vi "Create.vi"(8 "error in (no error)":errorcluster, 10 "Append Index (-1)":i32=-1, 11 "File Type":T1) -> (0 "error out":errorcluster, 3 "Data out":refnum<class "Data.lvclass">)   [LabVIEW 2019, in "Data.lvclass"]
uses:
  Data.lvclass
  Data.DAT/Data.DAT.lvclass
  Data.ITX/Data.ITX.lvclass
  Data.TDMS/Data.TDMS.lvclass
  Typedefs/File Type--enum.ctl
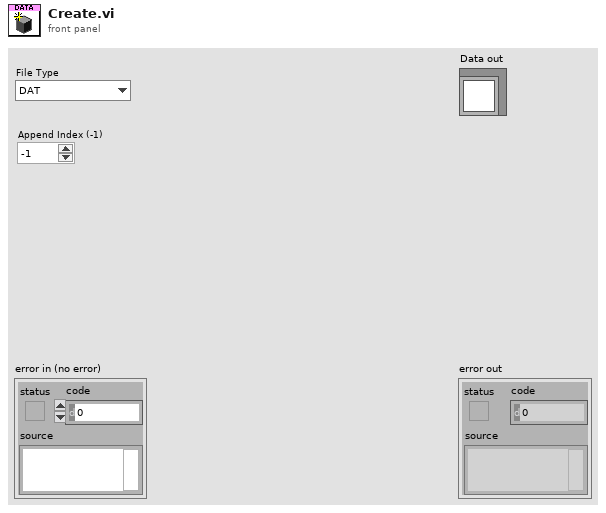
[diagram p1: front panel]
types:
  T1 = typedef "Data.lvclass/File Type--enum.ctl" = enum16{"DAT", "ITX", "TDMS", "VI"}
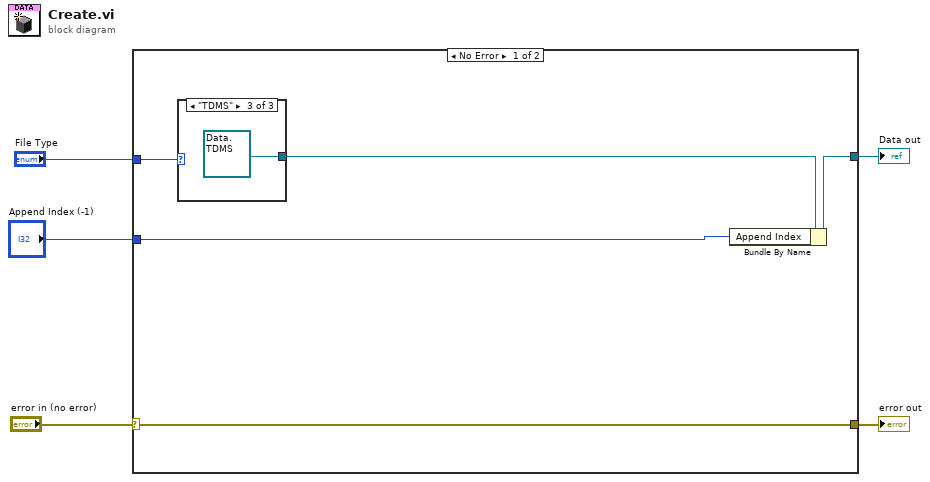
[diagram p0: block diagram]
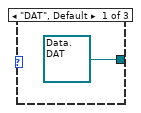
[diagram p2: hidden frame]
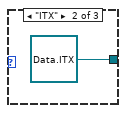
[diagram p3: hidden frame]
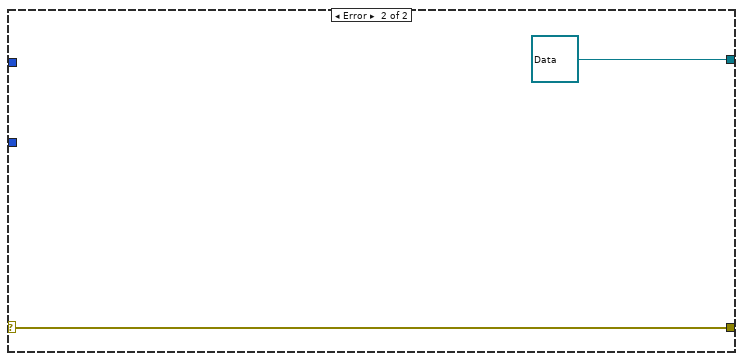
[diagram p4: hidden frame]
diagram:
  n1 = case shown="No Error" "error in (no error)" {
    selector: "error in (no error)" -> [w10 w15]
    tunnel: [w10 w15] -> w4
    tunnel: [w7 refnum<class "Data.lvclass"> refnum ("ITX")] -> w3
    tunnel: "File Type" -> [w9 _]
    tunnel: "Append Index (-1)" -> [w6 _]
    frame No Error {
      n2 = case shown="\"TDMS\"" w9 {
        tunnel: [refnum<class "Data.DAT.lvclass"> refnum ("DAT.lvclass") refnum<class "Data.ITX.lvclass"> refnum ("ITX") refnum<class "Data.TDMS.lvclass"> refnum ("Data.TDMS.lvclass")] -> w8
        frame "DAT", Default {
        }
        frame "ITX" {
        }
        frame "TDMS" {
        }
      }
      n3 = Bundle By Name(cluster=w8, "Append Index"=w6) -> (w7:refnum<class "Data.lvclass">)
    }
    frame Error {
    }
  }
  "error out" <- w4
  "Data out" <- w3
